vi "Expose.vi"(0 "Url":string, 1 "Register for events (T)":bool=TRUE, 2 "EventsCategory":string caption="Events Category", 5 "Create Handler":refnum<vi>, 7 "Destroy Handler":refnum<vi>, 9 "Invoke Method":refnum<vi>, 12 "DoLogging":bool, 13 "Timeout (ms)":i32) -> (4 "Expose":T1)   [LabVIEW 2017]
uses:
  ExposeInfo.ctl
  C:/Code/CMCryoSysCode/Expose/COM/CSCom/CSCom/bin/Release/CSCom.dll
  COM/CSCom/CSCom/bin/Release/CSCom.dll
  ExposeHandlers.ctl
  ExposeMessageCallbackInfo.ctl
panel:
  out "error out":errorcluster
  in  "error in (no error)":errorcluster
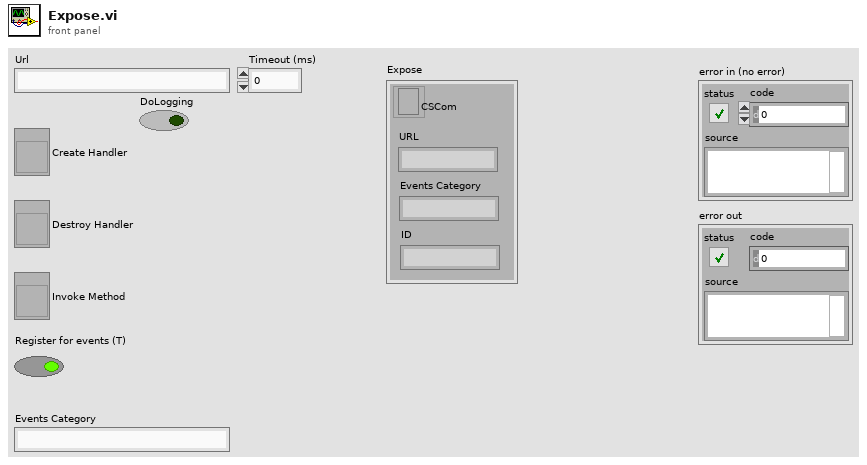
[diagram p1: front panel]
types:
  T1 = typedef "ExposeInfo.ctl" = cluster{"CSCom":refnum<k24>, "URL":string, "Events Category":string, "ID":string}
  T2 = typedef "ExposeHandlers.ctl" = cluster{"Create":refnum<vi>, "Destroy":refnum<vi>, "Invoke":refnum<vi>, "Get":refnum<vi>, "Set":refnum<vi>, "Error":refnum<vi>, "Warning":refnum<vi>}
  T3 = typedef "ExposeMessageCallbackInfo.ctl" = cluster{"Expose Info":T1, "Expose Handlers":T2}
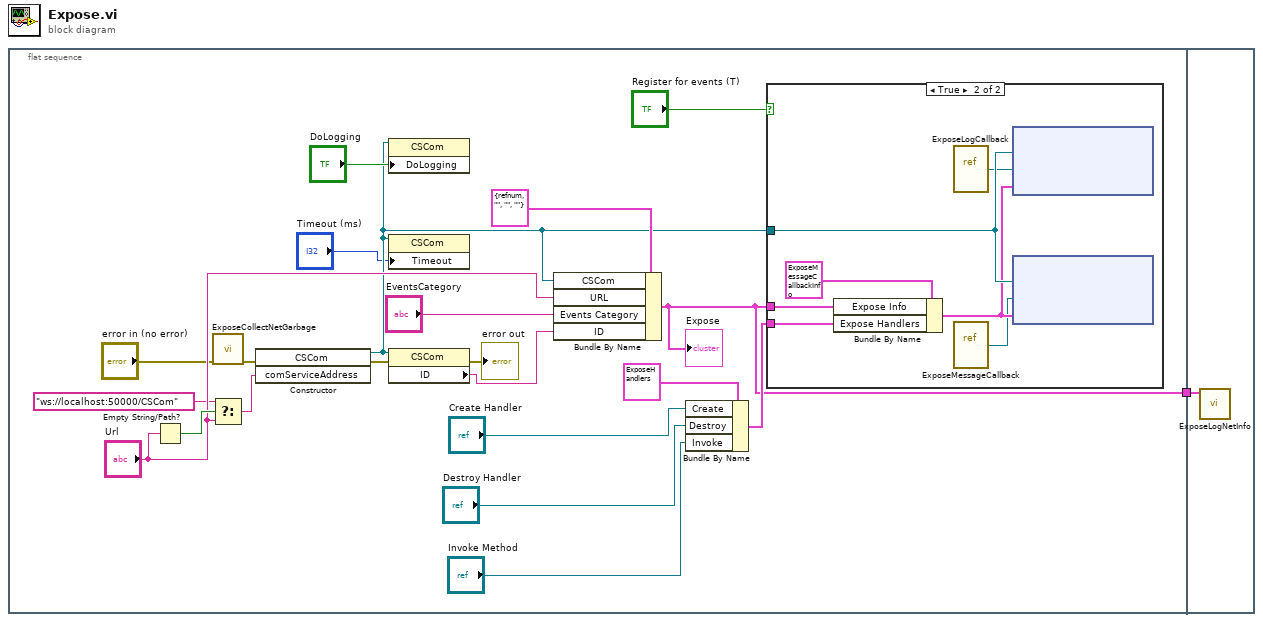
[diagram p0: block diagram]
diagram:
  n1 = flat-sequence {
    tunnel: [w5] -> w1
    tunnel: w1 -> [w30]
    frame #0 {
      n2 = Empty String/Path?(string/path="Url") -> (empty?=w12:bool)
      n3 = call "ExposeCollectNetGarbage.vi"("error in (no error)"="error in (no error)") -> ("error out"=w7:errorcluster)  [unwired: 10 in]
      n4 = Select(t="ws://localhost:50000/CSCom" ("comServiceAddress"), s=w12, f="Url") -> (s? t:f=w9:string)
      n5 = constructor class="CSCom"(error in=w7, "comServiceAddress"=w9) -> (reference out=w3:refnum<k24>, error out=w6:errorcluster)  [unwired: 2 in, 2 out]
      n6 = property class="CSCom"(reference=w3, "DoLogging"="DoLogging") -> ()  [unwired: 1 in, 2 out]
      n7 = property class="CSCom"(reference=w3, "Timeout"="Timeout (ms)") -> ()  [unwired: 1 in, 2 out]
      n8 = property class="CSCom"(reference=w3, error in=w6) -> (error out=→"error out":errorcluster, "ID"=w14:string)  [unwired: 1 out]
      n9 = Bundle By Name(cluster=T1 {"CSCom"=refnum, "URL"="", "Events Category"="", "ID"=""} ("Handler Info"), "CSCom"=w3, "URL"="Url", "Events Category"="EventsCategory", "ID"=w14) -> (w5:T1)
      "Expose" <- w5
      n10 = Bundle By Name(cluster=T2 {"Create"=refnum, "Destroy"=refnum, "Invoke"=refnum, "Get"=refnum, "Set"=refnum, "Error"=refnum, "Warning"=refnum} ("Expose Handlers"), "Create"="Create Handler", "Destroy"="Destroy Handler", "Invoke"="Invoke Method") -> (w15:T2)
      n11 = case shown="True" "Register for events (T)" {
        tunnel: w3 -> [_ w29]
        tunnel: w5 -> [_ w27]
        tunnel: w15 -> [_ w26]
        frame False {
        }
        frame True {
          n12 = Bundle By Name(cluster=T3 {"Expose Info"={"CSCom"=refnum, "URL"="", "Events Category"="", "ID"=""}, "Expose Handlers"={"Create"=refnum, "Destroy"=refnum, "Invoke"=refnum, "Get"=refnum, "Set"=refnum, "Error"=refnum, "Warning"=refnum}}, "Expose Info"=w27, "Expose Handlers"=w26) -> (w25:T3)
          n13 = vi-ref "ExposeLogCallback.vi"() -> ("vi reference"=w24:refnum<vi>)
          n14 = vi-ref "ExposeMessageCallback.vi"() -> ("vi reference"=w23:refnum<vi>)
          n15 = node(w29, w24, w25) -> ()  [unwired: 2 in, 2 out]
          n16 = node(w29, w23, w25) -> ()  [unwired: 2 in, 2 out]
        }
      }
    }
    frame #1 {
      n17 = call "ExposeLogNetInfo.vi"("Expose Info"=w30) -> ()  [unwired: 11 in]
    }
  }
